vi "Show Hide Avg Fuel.vi"(0 "Bool":bool, 1 "Reference Cluster":T1) -> ()   [LabVIEW 2017, in "GUI.lvlib"]
uses:
  GUI.lvlib
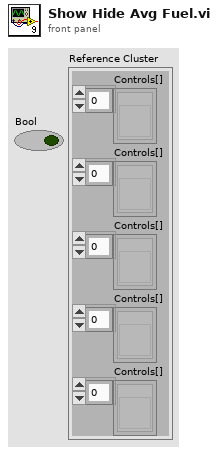
[diagram p1: front panel]
types:
  T1 = cluster{"Controls[]":refnum<vi>[], "Controls[]":refnum<vi>[], "Controls[]":refnum<vi>[], "Controls[]":refnum<vi>[], "Controls[]":refnum<vi>[]}
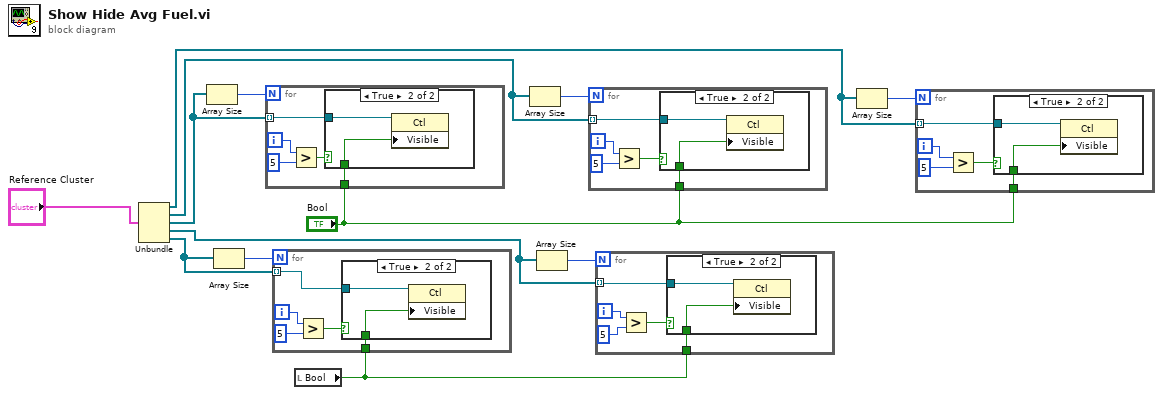
[diagram p0: block diagram]
diagram:
  n1 = Unbundle("Reference Cluster") -> ("Controls[]"=w5:refnum<vi>[], "Controls[]"=w4:refnum<vi>[], "Controls[]"=w3:refnum<vi>[], "Controls[]"=w1:refnum<vi>[], "Controls[]"=w2:refnum<vi>[])
  n2 = Array Size(array=w3) -> (size(s)=w13:i32)
  n3 = Array Size(array=w2) -> (size(s)=w10:i32)
  n4 = for {
    N: w13 -> [_]
    tunnel: w3 -> [w15] mode=indexing
    tunnel: "Bool" -> [w14]
    i -> [w18]
    n5 = Greater?(x=w18, y=5) -> (0:w16:bool)
    n6 = case shown="True" w16 {
      tunnel: w15 -> [_ w20]
      tunnel: w14 -> [_ w19]
      frame False {
      }
      frame True {
        n7 = property class="Ctl"(reference=w20, "Visible"=w19) -> ()  [unwired: 1 in, 2 out]
      }
    }
  }
  n8 = local read "Bool"() -> (w7:bool)
  n9 = for {
    N: w10 -> [_]
    tunnel: w2 -> [w23] mode=indexing
    tunnel: w7 -> [w21]
    i -> [w25]
    n10 = Greater?(x=w25, y=5) -> (0:w22:bool)
    n11 = case shown="True" w22 {
      tunnel: w23 -> [_ w27]
      tunnel: w21 -> [_ w26]
      frame False {
      }
      frame True {
        n12 = property class="Ctl"(reference=w27, "Visible"=w26) -> ()  [unwired: 1 in, 2 out]
      }
    }
  }
  n13 = Array Size(array=w4) -> (size(s)=w12:i32)
  n14 = Array Size(array=w1) -> (size(s)=w9:i32)
  n15 = for {
    N: w12 -> [_]
    tunnel: w4 -> [w29] mode=indexing
    tunnel: "Bool" -> [w28]
    i -> [w32]
    n16 = Greater?(x=w32, y=5) -> (0:w30:bool)
    n17 = case shown="True" w30 {
      tunnel: w29 -> [_ w34]
      tunnel: w28 -> [_ w33]
      frame False {
      }
      frame True {
        n18 = property class="Ctl"(reference=w34, "Visible"=w33) -> ()  [unwired: 1 in, 2 out]
      }
    }
  }
  n19 = for {
    N: w9 -> [_]
    tunnel: w1 -> [w36] mode=indexing
    tunnel: w7 -> [w35]
    i -> [w39]
    n20 = Greater?(x=w39, y=5) -> (0:w37:bool)
    n21 = case shown="True" w37 {
      tunnel: w36 -> [_ w41]
      tunnel: w35 -> [_ w40]
      frame False {
      }
      frame True {
        n22 = property class="Ctl"(reference=w41, "Visible"=w40) -> ()  [unwired: 1 in, 2 out]
      }
    }
  }
  n23 = Array Size(array=w5) -> (size(s)=w11:i32)
  n24 = for {
    N: w11 -> [_]
    tunnel: w5 -> [w43] mode=indexing
    tunnel: "Bool" -> [w42]
    i -> [w44]
    n25 = Greater?(x=w44, y=5) -> (0:w45:bool)
    n26 = case shown="True" w45 {
      tunnel: w43 -> [_ w48]
      tunnel: w42 -> [_ w47]
      frame False {
      }
      frame True {
        n27 = property class="Ctl"(reference=w48, "Visible"=w47) -> ()  [unwired: 1 in, 2 out]
      }
    }
  }
